vi "Obtain Experimental Queue.vi"() -> (0 "Queue":T1)   [LabVIEW 2013]
uses:
  test/Runtime/Sidecar Debug Queue.ctl
  Experimental Configuration.ctl
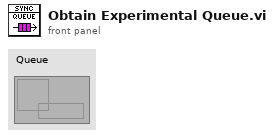
[diagram p1: front panel]
types:
  T1 = typedef "Sidecar Debug Queue.ctl" = refnum<queue>
  T2 = typedef "Runtime Queue.ctl" = refnum<queue>
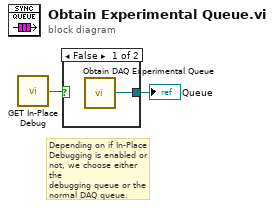
[diagram p0: block diagram]
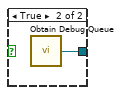
[diagram p2: hidden frame]
diagram:
  # "Depending on if In-Place\nDebugging is enabled or\nnot, we choose either the\ndebugging queue or the\nnormal DAQ queue."
  n1 = call "GET In-Place Debug.vi"() -> ("In Place Debug Enabled"=w2:bool)
  n2 = case shown="False" w2 {
    tunnel: [w3 w4] -> w1
    frame False {
      n3 = call "Obtain DAQ Experimental Queue.vi"() -> ("Experimental DAQ Queue"=w3:T2)
    }
    frame True {
      n4 = call "Obtain Debug Queue.vi"() -> ("Debug Queue"=w4:T1)
    }
  }
  "Queue" <- w1
